vi "Read tdms file ref.vi"(8 "error in (no error)":errorcluster, 11 "TDMS in":refnum<class "TDMS.lvclass">) -> (0 "error out":errorcluster, 2 "tdms file ref":refnum<k34>, 3 "TDMS out":refnum<class "TDMS.lvclass">)   [LabVIEW 2019, in "ManejoArchivos.lvlib" / "TDMS.lvclass"]
uses:
  TDMS.lvclass
  TDMS.lvclass/TDMS.ctl
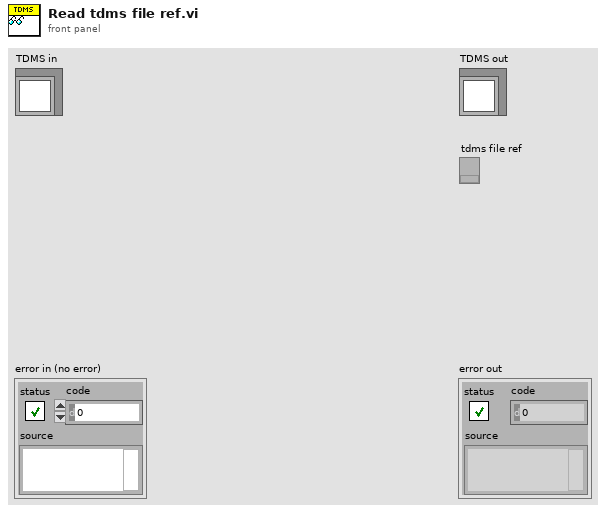
[diagram p1: front panel]
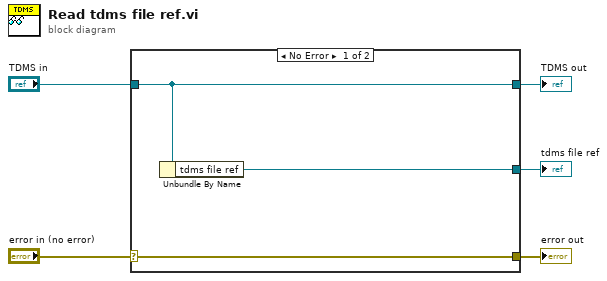
[diagram p0: block diagram]
diagram:
  n1 = case shown="No Error" "error in (no error)" {
    selector: "error in (no error)" -> [w8 w9]
    tunnel: [w8 w9] -> w4
    tunnel: [w7 w10] -> w2
    tunnel: "TDMS in" -> [w7 w10]
    tunnel: [w6 _] -> w1
    frame No Error {
      n2 = Unbundle By Name(w7) -> ("tdms file ref"=w6:refnum<k34>)
    }
    frame Error {
    }
  }
  "error out" <- w4
  "TDMS out" <- w2
  "tdms file ref" <- w1
